vi "RPC Method PerformACIRMeasurement.vi"(8 "error in (no error)":errorcluster, 11 "OOP Server in":refnum<class "OCV2.lvclass">) -> (0 "error out":errorcluster, 3 "OOP Server out":refnum<class "OCV2.lvclass">)   [LabVIEW 2019, in "OCV2.lvlib" / "OCV2.lvclass"]
uses:
  OCV2.lvclass
  OCV2.lvclass/OCV2.ctl
  RPC Messages/measurementservice_ErrorOut/measurementservice_ErrorOut_Data.ctl
  RPC Messages/measurementservice_ACIRData/measurementservice_ACIRData_Data.ctl
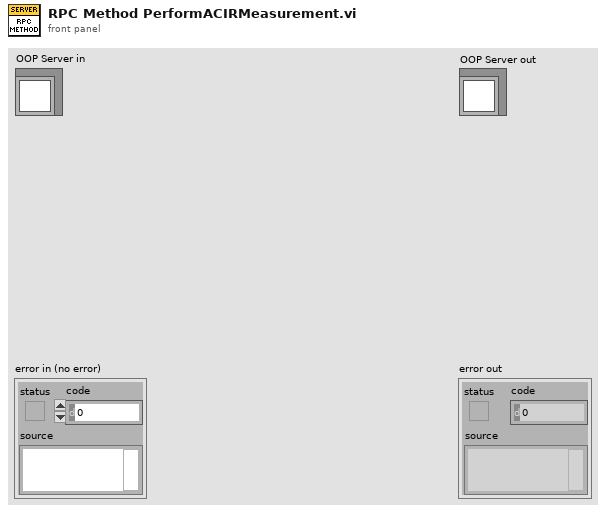
[diagram p1: front panel]
types:
  T1 = typedef "OCV2.lvlib/OCV2.lvclass/measurementservice_ErrorOut_Data.ctl" = cluster{"errCode":i32, "errMessage":string}
  T2 = typedef "OCV2.lvlib/OCV2.lvclass/measurementservice_ACIRData_Data.ctl" = cluster{"Impedance":sgl[], "Real":sgl[], "Imaginery":sgl[], "error":T1}
  T3 = typedef "OCV2.lvlib/OCV2.lvclass/Server Internal UEs.ctl" = cluster{"Invoke Internal UE":refnum<user-event>, "Query Internal UE":refnum<user-event>, "PerformOCVMeasurement Internal UE":refnum<user-event>, "PerformACIRMeasurement Internal UE":refnum<user-event>, "StreamOCVMeasurement Internal UE":refnum<user-event>, "Register Internal UE":refnum<user-event>}
  T4 = typedef "OCV2.lvlib/OCV2.lvclass/Server gRPC UEs.ctl" = cluster{"Invoke gRPC UE":refnum<user-event>, "Query gRPC UE":refnum<user-event>, "PerformOCVMeasurement gRPC UE":refnum<user-event>, "PerformACIRMeasurement gRPC UE":refnum<user-event>, "StreamOCVMeasurement gRPC UE":refnum<user-event>, "Register gRPC UE":refnum<user-event>}
  T5 = typedef "OCV2.lvlib/gprc-lvsupport.lvlib/grpcId.ctl" = u64
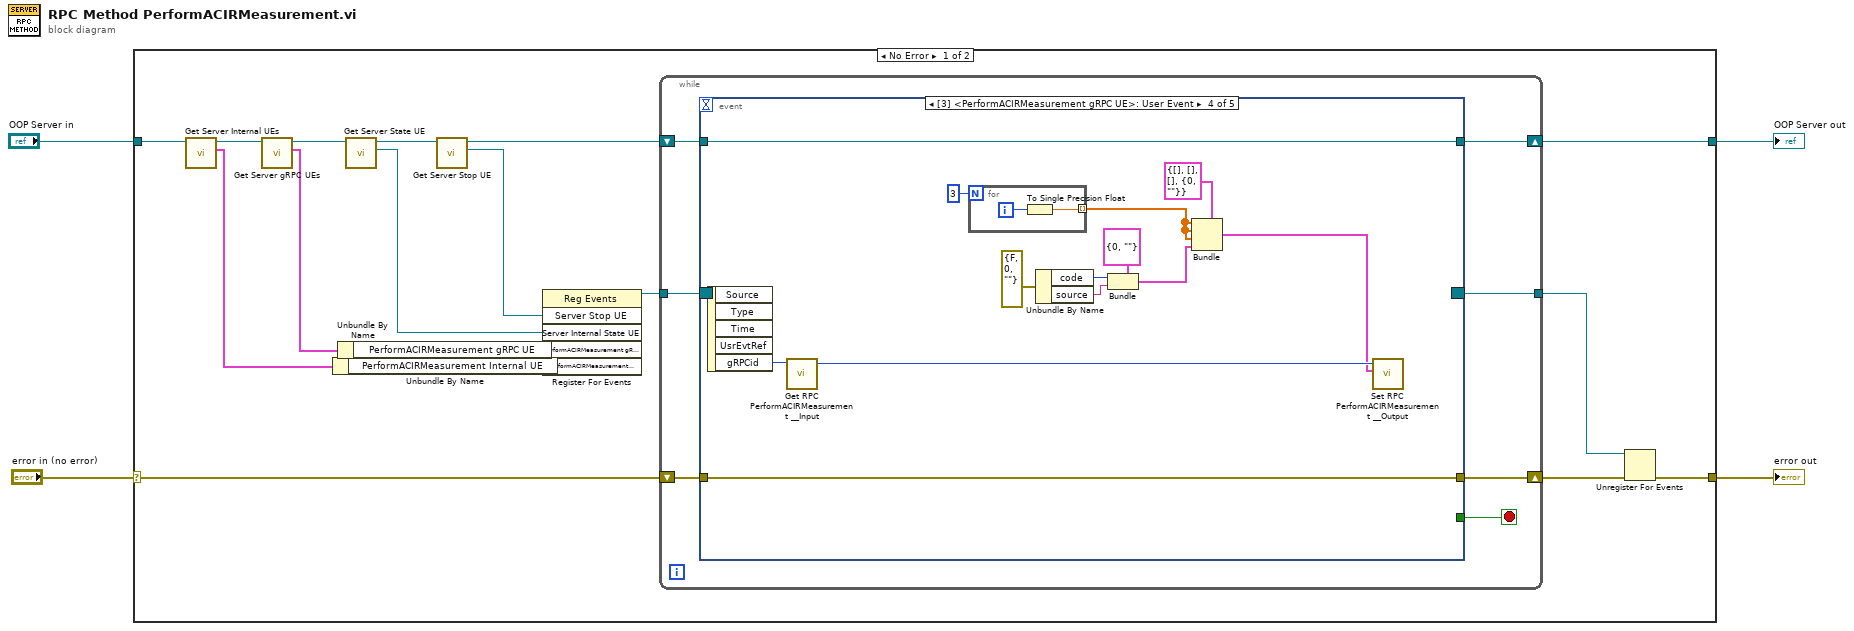
[diagram p0: block diagram]
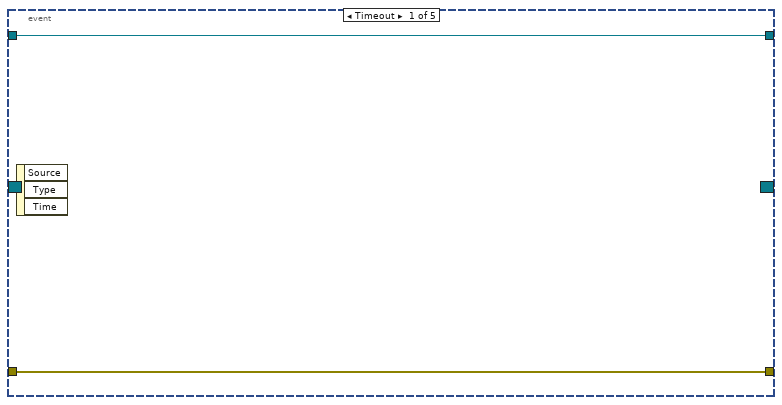
[diagram p2: hidden frame]
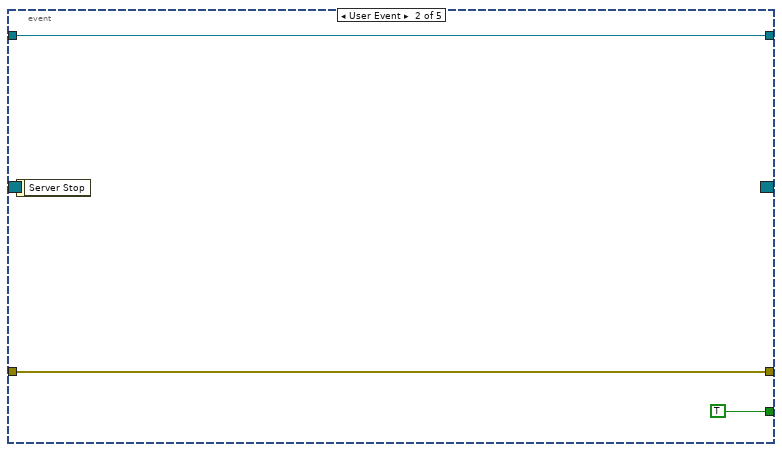
[diagram p3: hidden frame]
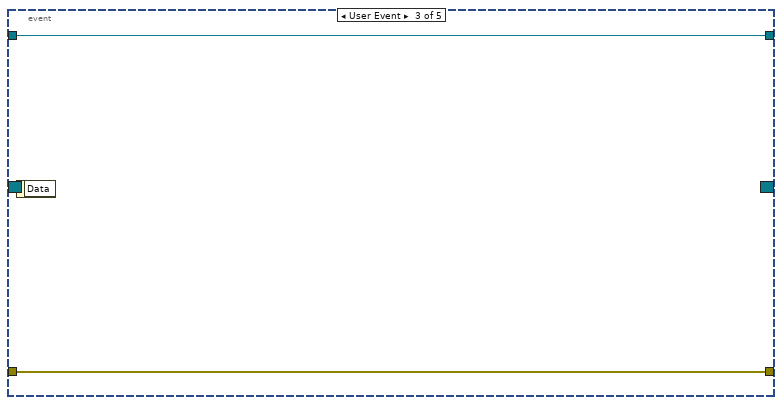
[diagram p4: hidden frame]
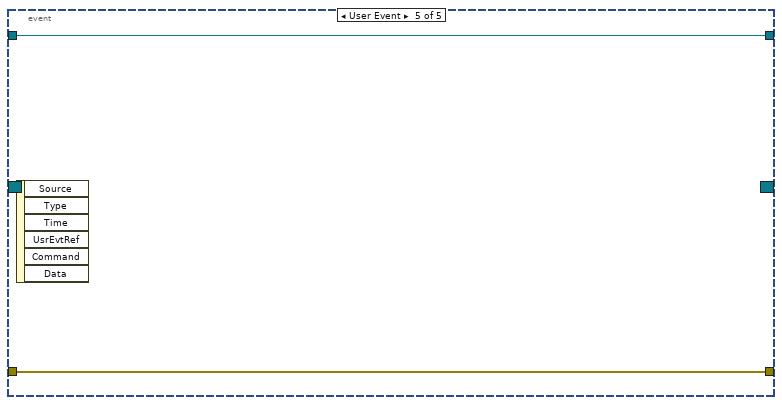
[diagram p5: hidden frame]
diagram:
  n1 = case shown="No Error" "error in (no error)" {
    selector: "error in (no error)" -> [w17 w54]
    tunnel: [w15 w54] -> w3
    tunnel: "OOP Server in" -> [w19 w53]
    tunnel: [w5 w53] -> w1
    frame No Error {
      n2 = call "Get Server Internal UEs.vi"("OOP Server in"=w19) -> ("Server Internal UEs"=w11:T3, "OOP Server out"=w18:refnum<class "OCV2.lvclass">)  [unwired: 9 in]
      n3 = call "Get Server gRPC UEs.vi"("OOP Server in"=w18) -> ("Server gRPC UEs"=w13:T4, "OOP Server out"=w8:refnum<class "OCV2.lvclass">)  [unwired: 9 in]
      n4 = Unbundle By Name ("Unbundle Internal UE")(w11) -> ("PerformACIRMeasurement Internal UE"=w10:refnum<user-event>)
      n5 = Unbundle By Name ("Unbundle gRPC UE")(w13) -> ("PerformACIRMeasurement gRPC UE"=w12:refnum<user-event>)
      n6 = call "Get Server State UE.vi"("Template Server in"=w8) -> ("Server Internal State UE"=w6:refnum<user-event>, "Template Server out"=w7:refnum<class "OCV2.lvclass">)  [unwired: 9 in]
      n7 = call "Get Server Stop UE.vi"("OOP Server in"=w7) -> ("Server Stop UE"=w21:refnum<user-event>, "OOP Server out"=w9:refnum<class "OCV2.lvclass">)  [unwired: 9 in]
      n8 = register-events(w21, w6, w12, w10) -> (reference out=w20:refnum<event-registration>)  [unwired: 2 in, 1 out]
      n9 = while {
        tunnel: w20 -> [w28]
        tunnel: [w24] -> w14
        shift-right: [w25] -> w16
        shift-left: w17 -> [w26]
        shift-right: [w22] -> w5
        shift-left: w9 -> [w23]
        stop <- w27 stop-if-true
        n10 = event "RPC Method Event Structure" shown="[3] <PerformACIRMeasurement gRPC UE>: User Event" {
          selector: w28 -> [_ _ _ _ _]
          dyn-events: [_ _ _ _ _] -> w24
          timeout: _ -> [_ _ _ _ _]
          tunnel: [_ TRUE _ _ _] -> w27
          tunnel: w26 -> [w30 w32 w35 w48 w52]
          tunnel: [w30 w32 w35 w48 w52] -> w25
          tunnel: w23 -> [w29 w31 w34 w47 w51]
          tunnel: [w29 w31 w34 w47 w51] -> w22
          event Timeout {
            n11 = event-data() -> ()  [unwired: 1 in, 3 out]
          }
          event User Event {
            n12 = event-data() -> ()  [unwired: 1 in, 1 out]
          }
          event User Event {
            n13 = event-data() -> ()  [unwired: 1 in, 1 out]
          }
          event User Event {
            n14 = event-data() -> ("gRPCid"=w46:T5)  [unwired: 1 in, 4 out]
            n15 = call "Get RPC PerformACIRMeasurement __Input.vi"("gRPCid in"=w46) -> ("gRPCid out"=w45:T5)  [unwired: 8 in, 2 out]
            n16 = for {
              N: 3 -> [_]
              tunnel: [w50] -> w38 mode=indexing
              i -> [w49]
              n17 = To Single Precision Float(number=w49) -> (single precision float=w50:sgl)
            }
            n18 = Unbundle By Name(errorcluster {"status"=FALSE, "code"=0, "source"=""} ("error in (no error)")) -> ("code"=w42:i32, "source"=w41:string)
            n19 = Bundle(cluster=T1 {"errCode"=0, "errMessage"=""} ("error"), "errCode"=w42, "errMessage"=w41) -> (w37:T1)
            n20 = Bundle(cluster=T2 {"Impedance"=[], "Real"=[], "Imaginery"=[], "error"={"errCode"=0, "errMessage"=""}} ("Message Data"), "Impedance"=w38, "Real"=w38, "Imaginery"=w38, "error"=w37) -> (w36:T2)
            n21 = call "Set RPC PerformACIRMeasurement __Output.vi"("Message Data"=w36, "gRPCid in"=w45) -> ()  [unwired: 9 in, 1 out]
          }
          event User Event {
            n22 = event-data() -> ()  [unwired: 1 in, 6 out]
          }
        }
      }
      n23 = Unregister For Events(event registration refnum=w14, error in=w16) -> (error out=w15:errorcluster)
    }
    frame Error {
    }
  }
  "error out" <- w3
  "OOP Server out" <- w1
